vi "英维克空调告警存储.vi"(11 "x+1":refnum<vi>) -> ()   [LabVIEW 2016, in "环境动力监测库.lvlib" / "空调库.lvlib"]
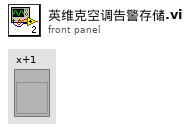
[diagram p1: front panel]
types:
  T1 = cluster{"型号选择":enum16{"黑盾", "英维克", "仁科测控RS-KTC-N01"}, "MB session in":refnum<class "MB_Master.lvclass">, "英维克空调寄存器":u16[], "通讯状态":bool, "PORT":string, "IP":string, "Slave ID ":u8, "Serial Config":cluster{"baud rate (bps)":u32, "stop bits":u16, "parity":u16, "flow control":u16, "timeout":u32, "retries":i32}, "VISA Resource":refnum<visa-resource-name>, "MB通信方式选择":enum16{"串口", "TCP"}}
  T2 = cluster{"高温告警":bool, "低温告警":bool, "高湿告警":bool, "低湿告警":bool, "盘管防冻":bool, "排气高温":bool, "盘管温感失效":bool, "室外温感失效":bool, "冷凝温感失效":bool, "内温感失效":bool, "排气温感失效":bool, "湿感失效":bool, "内风机故障":bool, "外风机故障":bool, "压缩机故障":bool, "电加热故障":bool, "应急风机故障":bool, "高压告警":bool, "低压告警":bool, "水浸告警":bool, "烟感告警":bool, "门禁告警":bool, "高压锁定":bool, "低压锁定":bool, "排气锁定":bool, "交流过压":bool, "交流欠压":bool, "交流掉压":bool, "缺相":bool, "频率异常":bool, "逆相":bool, "直流过压":bool, "直流欠压":bool}
  T3 = cluster{"漏水监测输出":cluster{"漏水监测告警":bool, "告警内容":string}, "门禁监测输出":cluster{"门禁监测告警":bool, "告警内容":string}, "门禁监测输出2":cluster{"门禁监测告警":bool, "告警内容":string}, "温湿度监测输出":cluster{"温湿度监测告警":bool, "告警内容":string}, "烟雾监测输出":cluster{"烟雾监测告警":bool, "告警内容":string}, "空调监测输出":cluster{"空调监测告警":bool, "告警内容":string}, "自动重合闸输出":cluster{"自动重合闸告警":bool, "告警内容":string}, "红外入侵输出":cluster{"红外入侵告警":bool, "告警内容":string}, "振动输出":cluster{"振动告警":bool, "告警内容":string}, "UPS输出":cluster{"UPS告警":bool, "告警内容":string}, "蓄电池输出":cluster{"蓄电池告警":bool, "告警内容":string}, "蓄电池输出2":cluster{"蓄电池告警":bool, "告警内容":string}, "GPS输出":cluster{"定位告警":bool, "告警内容":string}, "北斗输出":cluster{"定位告警":bool, "告警内容":string}, "气象输出":cluster{"气象告警":bool, "告警内容":string}}
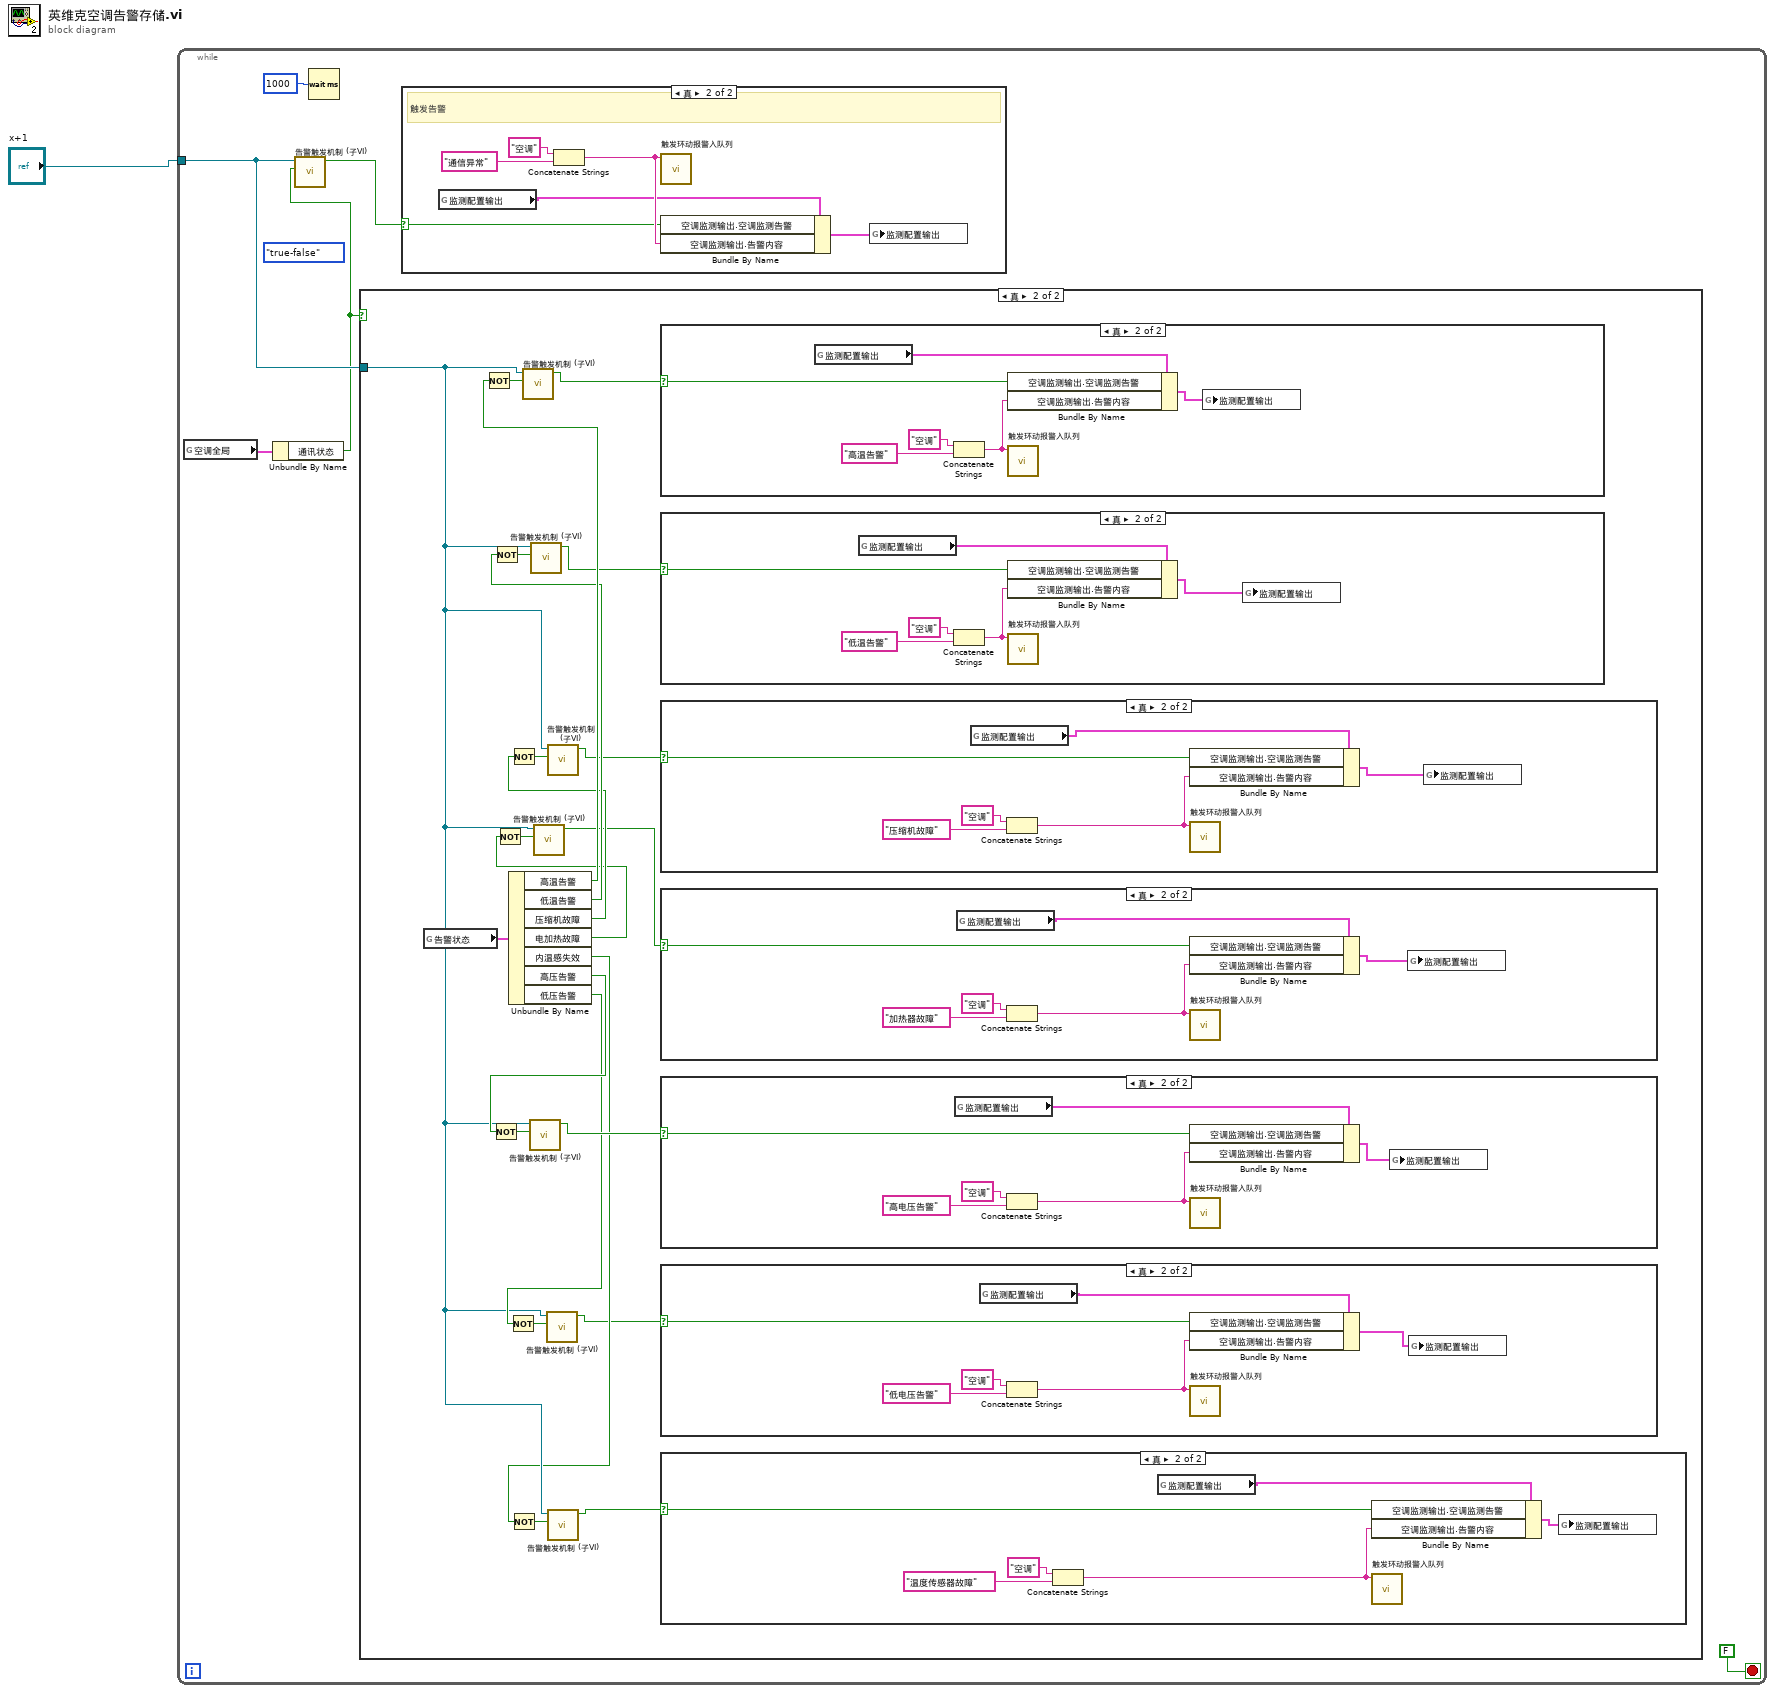
[diagram p0: block diagram]
diagram:
  n1 = while {
    tunnel: "x+1" -> [w4]
    stop <- FALSE stop-if-true
    (unwired) enum16{"either", "false-true", "true-false"}."true-false" ("direction")
    n2 = global read "断电保存全局变量.vi" "空调全局"() -> (w3:T1)
    n3 = Unbundle By Name(w3) -> ("通讯状态"=w2:bool)
    n4 = call "告警触发机制 (子VI).vi"("状态输出"=w2, "Digital输入"=w4) -> ("触发告警"=w5:bool)  [unwired: 8 in, 1 out]
    n5 = Wait (ms)(milliseconds to wait=u32 1000 ("等待时间（毫秒）")) -> ()  [unwired: 1 out]
    n6 = case shown="真" w2 {
      tunnel: w4 -> [_ w11]
      frame False {
      }
      frame True {
        n7 = global read "内部交互全局变量.vi" "告警状态"() -> (w30:T2)
        n8 = Unbundle By Name(w30) -> ("高温告警"=w27:bool, "低温告警"=w24:bool, "压缩机故障"=w22:bool, "电加热故障"=w19:bool, "内温感失效"=w10:bool, "高压告警"=w16:bool, "低压告警"=w12:bool)
        n9 = Not(x=w27) -> (.not. x?=w29:bool)
        n10 = Not(x=w16) -> (.not. x?=w17:bool)
        n11 = Not(x=w24) -> (.not. x?=w28:bool)
        n12 = Not(x=w19) -> (.not. x?=w20:bool)
        n13 = Not(x=w12) -> (.not. x?=w14:bool)
        n14 = Not(x=w22) -> (.not. x?=w25:bool)
        n15 = Not(x=w10) -> (.not. x?=w13:bool)
        n16 = call "告警触发机制 (子VI).vi"("状态输出"=w29, "Digital输入"=w11) -> ("触发告警"=w26:bool)  [unwired: 8 in, 1 out]
        n17 = call "告警触发机制 (子VI).vi"("状态输出"=w17, "Digital输入"=w11) -> ("触发告警"=w15:bool)  [unwired: 8 in, 1 out]
        n18 = call "告警触发机制 (子VI).vi"("状态输出"=w28, "Digital输入"=w11) -> ("触发告警"=w23:bool)  [unwired: 8 in, 1 out]
        n19 = call "告警触发机制 (子VI).vi"("状态输出"=w20, "Digital输入"=w11) -> ("触发告警"=w18:bool)  [unwired: 8 in, 1 out]
        n20 = call "告警触发机制 (子VI).vi"("状态输出"=w14, "Digital输入"=w11) -> ("触发告警"=w8:bool)  [unwired: 8 in, 1 out]
        n21 = call "告警触发机制 (子VI).vi"("状态输出"=w25, "Digital输入"=w11) -> ("触发告警"=w21:bool)  [unwired: 8 in, 1 out]
        n22 = call "告警触发机制 (子VI).vi"("状态输出"=w13, "Digital输入"=w11) -> ("触发告警"=w9:bool)  [unwired: 8 in, 1 out]
        n23 = case shown="真" w26 {
          selector: w26 -> [_ w66]
          frame False {
          }
          frame True {
            n24 = global read "内部交互全局变量.vi" "监测配置输出"() -> (w62:T3)
            n25 = Concatenate Strings("空调" ("设备"), "高温告警" ("日志信息")) -> (w63:string)
            n26 = Bundle By Name(cluster=w62, "空调监测输出.空调监测告警"=w66, "空调监测输出.告警内容"=w63) -> (w61:T3)
            n27 = call "触发环动报警入队列.vi"("报警内容"=w63) -> ()  [unwired: 11 in]
            n28 = global write "内部交互全局变量.vi" "监测配置输出"(w61) -> ()
          }
        }
        n29 = case shown="真" w23 {
          selector: w23 -> [_ w60]
          frame False {
          }
          frame True {
            n30 = global read "内部交互全局变量.vi" "监测配置输出"() -> (w56:T3)
            n31 = Concatenate Strings("空调" ("设备"), "低温告警" ("日志信息")) -> (w57:string)
            n32 = Bundle By Name(cluster=w56, "空调监测输出.空调监测告警"=w60, "空调监测输出.告警内容"=w57) -> (w55:T3)
            n33 = call "触发环动报警入队列.vi"("报警内容"=w57) -> ()  [unwired: 11 in]
            n34 = global write "内部交互全局变量.vi" "监测配置输出"(w55) -> ()
          }
        }
        n35 = case shown="真" w21 {
          selector: w21 -> [_ w72]
          frame False {
          }
          frame True {
            n36 = global read "内部交互全局变量.vi" "监测配置输出"() -> (w68:T3)
            n37 = Concatenate Strings("空调" ("设备"), "压缩机故障" ("日志信息")) -> (w69:string)
            n38 = Bundle By Name(cluster=w68, "空调监测输出.空调监测告警"=w72, "空调监测输出.告警内容"=w69) -> (w67:T3)
            n39 = call "触发环动报警入队列.vi"("报警内容"=w69) -> ()  [unwired: 11 in]
            n40 = global write "内部交互全局变量.vi" "监测配置输出"(w67) -> ()
          }
        }
        n41 = case shown="真" w18 {
          selector: w18 -> [_ w54]
          frame False {
          }
          frame True {
            n42 = global read "内部交互全局变量.vi" "监测配置输出"() -> (w50:T3)
            n43 = Concatenate Strings("空调" ("设备"), "加热器故障" ("日志信息")) -> (w51:string)
            n44 = Bundle By Name(cluster=w50, "空调监测输出.空调监测告警"=w54, "空调监测输出.告警内容"=w51) -> (w49:T3)
            n45 = call "触发环动报警入队列.vi"("报警内容"=w51) -> ()  [unwired: 11 in]
            n46 = global write "内部交互全局变量.vi" "监测配置输出"(w49) -> ()
          }
        }
        n47 = case shown="真" w15 {
          selector: w15 -> [_ w42]
          frame False {
          }
          frame True {
            n48 = global read "内部交互全局变量.vi" "监测配置输出"() -> (w38:T3)
            n49 = Concatenate Strings("空调" ("设备"), "高电压告警" ("日志信息")) -> (w39:string)
            n50 = Bundle By Name(cluster=w38, "空调监测输出.空调监测告警"=w42, "空调监测输出.告警内容"=w39) -> (w37:T3)
            n51 = call "触发环动报警入队列.vi"("报警内容"=w39) -> ()  [unwired: 11 in]
            n52 = global write "内部交互全局变量.vi" "监测配置输出"(w37) -> ()
          }
        }
        n53 = case shown="真" w8 {
          selector: w8 -> [_ w36]
          frame False {
          }
          frame True {
            n54 = global read "内部交互全局变量.vi" "监测配置输出"() -> (w32:T3)
            n55 = Concatenate Strings("空调" ("设备"), "低电压告警" ("日志信息")) -> (w33:string)
            n56 = Bundle By Name(cluster=w32, "空调监测输出.空调监测告警"=w36, "空调监测输出.告警内容"=w33) -> (w31:T3)
            n57 = call "触发环动报警入队列.vi"("报警内容"=w33) -> ()  [unwired: 11 in]
            n58 = global write "内部交互全局变量.vi" "监测配置输出"(w31) -> ()
          }
        }
        n59 = case shown="真" w9 {
          selector: w9 -> [_ w48]
          frame False {
          }
          frame True {
            n60 = Concatenate Strings("空调" ("设备"), "温度传感器故障" ("日志信息")) -> (w45:string)
            n61 = global read "内部交互全局变量.vi" "监测配置输出"() -> (w44:T3)
            n62 = Bundle By Name(cluster=w44, "空调监测输出.空调监测告警"=w48, "空调监测输出.告警内容"=w45) -> (w43:T3)
            n63 = call "触发环动报警入队列.vi"("报警内容"=w45) -> ()  [unwired: 11 in]
            n64 = global write "内部交互全局变量.vi" "监测配置输出"(w43) -> ()
          }
        }
      }
    }
    n65 = case shown="真" w5 {
      selector: w5 -> [_ w75]
      frame False {
      }
      frame True {
        # "触发告警"
        n66 = global read "内部交互全局变量.vi" "监测配置输出"() -> (w74:T3)
        n67 = Concatenate Strings("空调" ("设备"), "通信异常" ("日志信息")) -> (w76:string)
        n68 = call "触发环动报警入队列.vi"("报警内容"=w76) -> ()  [unwired: 11 in]
        n69 = Bundle By Name(cluster=w74, "空调监测输出.空调监测告警"=w75, "空调监测输出.告警内容"=w76) -> (w73:T3)
        n70 = global write "内部交互全局变量.vi" "监测配置输出"(w73) -> ()
      }
    }
  }
